vi "Get Path Segments.vi"(8 "error in (no error)":errorcluster, 11 "URI in":refnum<class "URI.lvclass">) -> (0 "error out":errorcluster, 2 "Segments":string[](array[string]), 3 "URI out":refnum<class "URI.lvclass">)   [LabVIEW 2013, in "openURI.lvlib" / "URI.lvclass"]
uses:
  URI.lvclass
  URI.lvclass/URI.ctl
  components/path/URI-Component.Path.lvclass/URI-Component.Path.ctl
  components/path/URI-Component.Path.lvclass
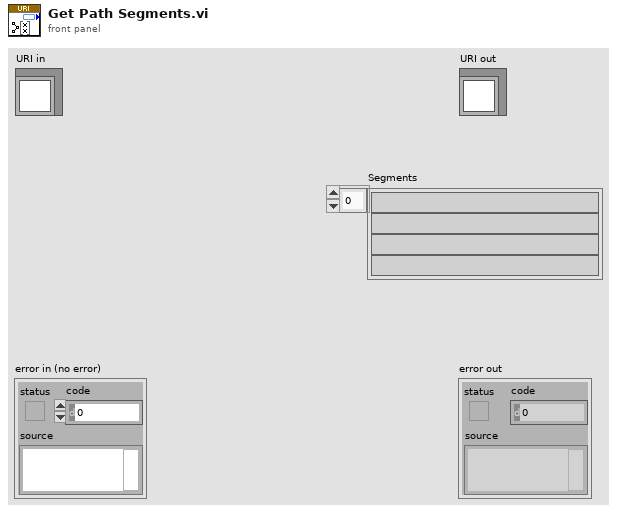
[diagram p1: front panel]
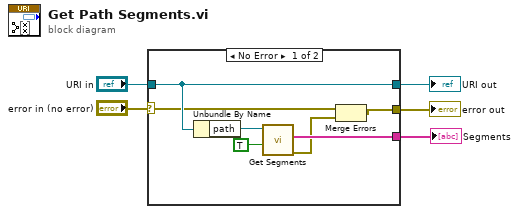
[diagram p0: block diagram]
diagram:
  n1 = case shown="No Error" "error in (no error)" {
    selector: "error in (no error)" -> [w11 w14]
    tunnel: [w10 w14] -> w4
    tunnel: [w12 w13] -> w2
    tunnel: "URI in" -> [w12 w13]
    tunnel: [w7 _] -> w1
    frame No Error {
      n2 = Unbundle By Name(w12) -> ("path"=w8:refnum<class "URI-Component.Path.lvclass">)
      n3 = call "Get Segments.vi"("Pct-Encoded? (F)"=TRUE ("Encoded? (F)"), "URI-Component.Path in"=w8) -> ("error out"=w6:errorcluster, "Segments"=w7:string[])  [unwired: 7 in, 1 out]
      n4 = Merge Errors(w11, w6) -> (w10:errorcluster)
    }
    frame Error {
    }
  }
  "error out" <- w4
  "URI out" <- w2
  "Segments" <- w1
